vi "Init.vi"(8 "error in (no error)":errorcluster, 9 "ConfigurationJSON":string="{\"VoltageLimit\":0,\"CurrentLimit\":0,\"UVP\":0,\"OVP\":15,\"Output Power On Mode (0: Safe)\":0,\"Overcurrent Protection Limit (0)\":1}", 10 "Address":string, 11 "RMX4120 in":refnum<class "RMX4120.lvclass">) -> (0 "error out":errorcluster, 1 "RunningInformation":string, 2 "Status":i32, 3 "RMX4120 out":refnum<class "RMX4120.lvclass">, 4 "ErrorCode":i32)   [LabVIEW 2023, in "RMX4120.lvclass"]
uses:
  RMX4120.lvclass
  RMX4120.lvclass/RMX4120.ctl
  Plugin/BLS Power Supply Template/RMX41xx_Config.ctl
  RMXPowerSupply.lvclass
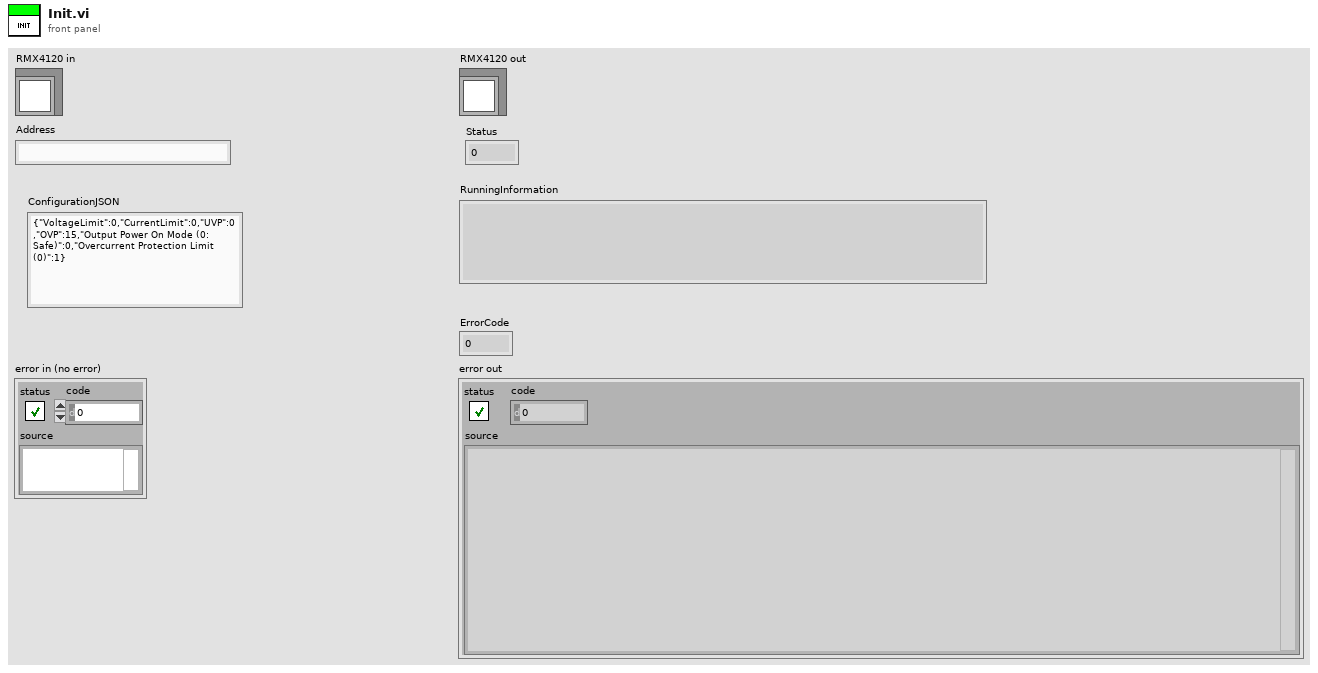
[diagram p1: front panel]
types:
  T1 = typedef "RMX41xx_Config.ctl" = cluster{"VoltageLimit":dbl, "CurrentLimit":dbl, "UVP":dbl, "OVP":dbl, "Output Power On Mode (0: Safe)":u16, "Overcurrent Protection Limit (0)":dbl}
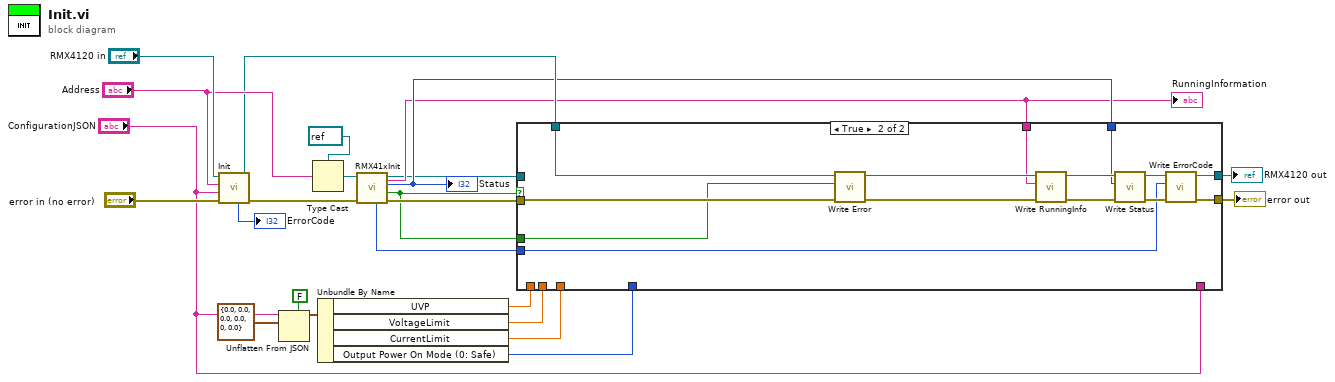
[diagram p0: block diagram]
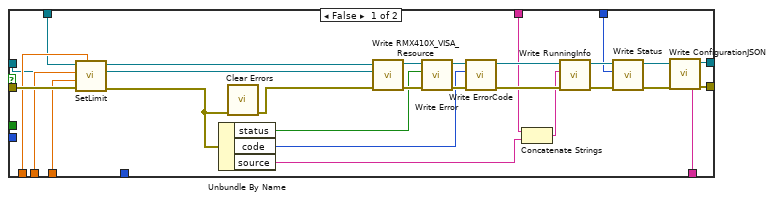
[diagram p2: hidden frame]
diagram:
  n1 = call-parent "Init.vi"("error in (no error)"="error in (no error)", "ConfigurationJSON"="ConfigurationJSON", "Address"="Address", "RMXPowerSupply in"="RMX4120 in") -> ("error out"=w18:errorcluster, "RMXPowerSupply out"=w17:refnum<class "RMX4120.lvclass">, "ErrorCode"=→"ErrorCode":i32)  [unwired: 3 in, 2 out]
  n2 = Unflatten From JSON(enable LabVIEW extensions? (T)=FALSE, JSON string="ConfigurationJSON", type and defaults=T1 {"VoltageLimit"=0.0, "CurrentLimit"=0.0, "UVP"=0.0, "OVP"=0.0, "Output Power On Mode (0: Safe)"=0, "Overcurrent Protection Limit (0)"=0.0} ("RMXPowerSupplyConfiguration")) -> (value=w6:T1)  [unwired: 4 in, 1 out]
  n3 = Type Cast(type=refnum<visa-resource-name> refnum ("VISA resource name"), x="Address") -> (*(type *) &x=w19:refnum<visa-resource-name>)
  n4 = Unbundle By Name(w6) -> ("UVP"=w1:dbl, "VoltageLimit"=w5:dbl, "CurrentLimit"=w4:dbl, "Output Power On Mode (0: Safe)"=w3:u16)
  n5 = call "RMX41xInit.vi"("VISA resource name"=w19, "error in (no error)"=w18) -> ("resulting string"=w12:string, "DeviceErrorCode"=w16:i32, "VISA resource name out"=w10:refnum<visa-resource-name>, "Status"=w15:i32, "Error"=w2:bool, "error out 2"=w11:errorcluster)  [unwired: 3 in]
  "RunningInformation" <- w12
  "Status" <- w15
  n6 = case shown="True" w2 {
    tunnel: w17 -> [w28 w65]
    tunnel: w2 -> [_ w55]
    tunnel: w16 -> [_ w56]
    tunnel: w15 -> [w29 w53]
    tunnel: [w43 w60] -> w14
    tunnel: [w41 w57] -> w13
    tunnel: w12 -> [w33 w54]
    tunnel: w11 -> [w40 w66]
    tunnel: w10 -> [w26 _]
    tunnel: "ConfigurationJSON" -> [w39 _]
    tunnel: w5 -> [w38 _]
    tunnel: w4 -> [w37 _]
    tunnel: w3 -> [_ _]
    tunnel: w1 -> [w36 _]
    frame False {
      n7 = call "SetLimit.vi"("Low Voltage Limit (0)"=w36, "error in (no error)"=w40, "Overcurrent Protection Limit (0)"=w37, "Overvoltage Protection Limit (0)"=w38, "RMXPowerSupply in"=w28) -> ("error out"=w25:errorcluster, "RMXPowerSupply out"=w27:refnum<class "RMX4120.lvclass">)  [unwired: 5 in]
      n8 = Unbundle By Name(w25) -> ("status"=w30:bool, "code"=w34:i32, "source"=w32:string)
      n9 = call <vilib>:"Clear Errors.vi"("error in (no error)"=w25) -> ("error out"=w35:errorcluster)  [unwired: 5 in, 1 out]
      n10 = call-dynamic "Write RMX410X_VISA_Resource.vi"("error in (no error)"=w35, "RMX410X_VISA_Resource"=w26, "RMXPowerSupply in"=w27) -> ("error out"=w51:errorcluster, "RMXPowerSupply out"=w52:refnum<class "RMX4120.lvclass">)  [unwired: 7 in]
      n11 = call-dynamic "Write Error.vi"("error in (no error)"=w51, "Error"=w30, "RMXPowerSupply in"=w52) -> ("error out"=w49:errorcluster, "RMXPowerSupply out"=w50:refnum<class "RMX4120.lvclass">)  [unwired: 7 in]
      n12 = call-dynamic "Write ErrorCode.vi"("error in (no error)"=w49, "ErrorCode"=w34, "RMXPowerSupply in"=w50) -> ("error out"=w47:errorcluster, "RMXPowerSupply out"=w48:refnum<class "RMX4120.lvclass">)  [unwired: 7 in]
      n13 = Concatenate Strings(w33, w32) -> (w31:string)
      n14 = call-dynamic "Write RunningInfo.vi"("error in (no error)"=w47, "RunningInfo"=w31, "RMXPowerSupply in"=w48) -> ("error out"=w45:errorcluster, "RMXPowerSupply out"=w46:refnum<class "RMX4120.lvclass">)  [unwired: 7 in]
      n15 = call-dynamic "Write Status.vi"("error in (no error)"=w45, "Status"=w29, "RMXPowerSupply in"=w46) -> ("error out"=w44:errorcluster, "RMXPowerSupply out"=w42:refnum<class "RMX4120.lvclass">)  [unwired: 7 in]
      n16 = call-dynamic "Write ConfigurationJSON.vi"("error in (no error)"=w44, "ConfigurationJSON"=w39, "RMXPowerSupply in"=w42) -> ("error out"=w43:errorcluster, "RMXPowerSupply out"=w41:refnum<class "RMX4120.lvclass">)  [unwired: 7 in]
    }
    frame True {
      n17 = call-dynamic "Write Error.vi"("error in (no error)"=w66, "Error"=w55, "RMXPowerSupply in"=w65) -> ("error out"=w63:errorcluster, "RMXPowerSupply out"=w64:refnum<class "RMX4120.lvclass">)  [unwired: 7 in]
      n18 = call-dynamic "Write RunningInfo.vi"("error in (no error)"=w63, "RunningInfo"=w54, "RMXPowerSupply in"=w64) -> ("error out"=w62:errorcluster, "RMXPowerSupply out"=w59:refnum<class "RMX4120.lvclass">)  [unwired: 7 in]
      n19 = call-dynamic "Write Status.vi"("error in (no error)"=w62, "Status"=w53, "RMXPowerSupply in"=w59) -> ("error out"=w61:errorcluster, "RMXPowerSupply out"=w58:refnum<class "RMX4120.lvclass">)  [unwired: 7 in]
      n20 = call-dynamic "Write ErrorCode.vi"("error in (no error)"=w61, "ErrorCode"=w56, "RMXPowerSupply in"=w58) -> ("error out"=w60:errorcluster, "RMXPowerSupply out"=w57:refnum<class "RMX4120.lvclass">)  [unwired: 7 in]
    }
  }
  "error out" <- w14
  "RMX4120 out" <- w13
